vi "dataMerge.vi"(8 "error in (no error)":errorcluster, 10 "data":string[][][](array[string]), 11 "reference in":refnum<class "File Controller.lvclass">) -> (0 "error out":errorcluster, 3 "reference out":refnum<class "File Controller.lvclass">)   [LabVIEW 2015, in "File Controller.lvclass"]
uses:
  File Controller.lvclass
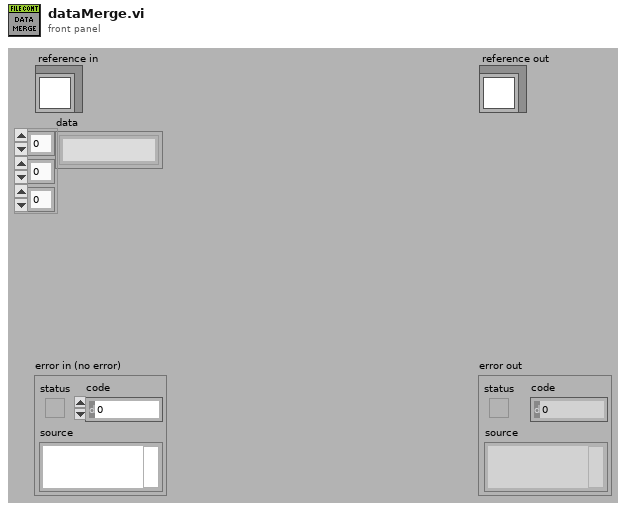
[diagram p1: front panel]
types:
  T1 = typedef "File Controller.lvclass/ObjectAttributesRef.ctl" = refnum<data-value>
  T2 = typedef "File Controller.lvclass/ObjectAttributes.ctl" = cluster{"MyAttribute":dbl, "file_path":path, "file_type":T3, "data":string[][][], "excel_file_ref":refnum<class "excelFile.lvclass">, "sheetName":string[], "subject_refs":refnum<class "subject.lvclass">[], "temp_data":string[][][]}
  T3 = typedef "excelFile.lvclass/fileType.ctl" = enum16{"database", "CosmedTest"}
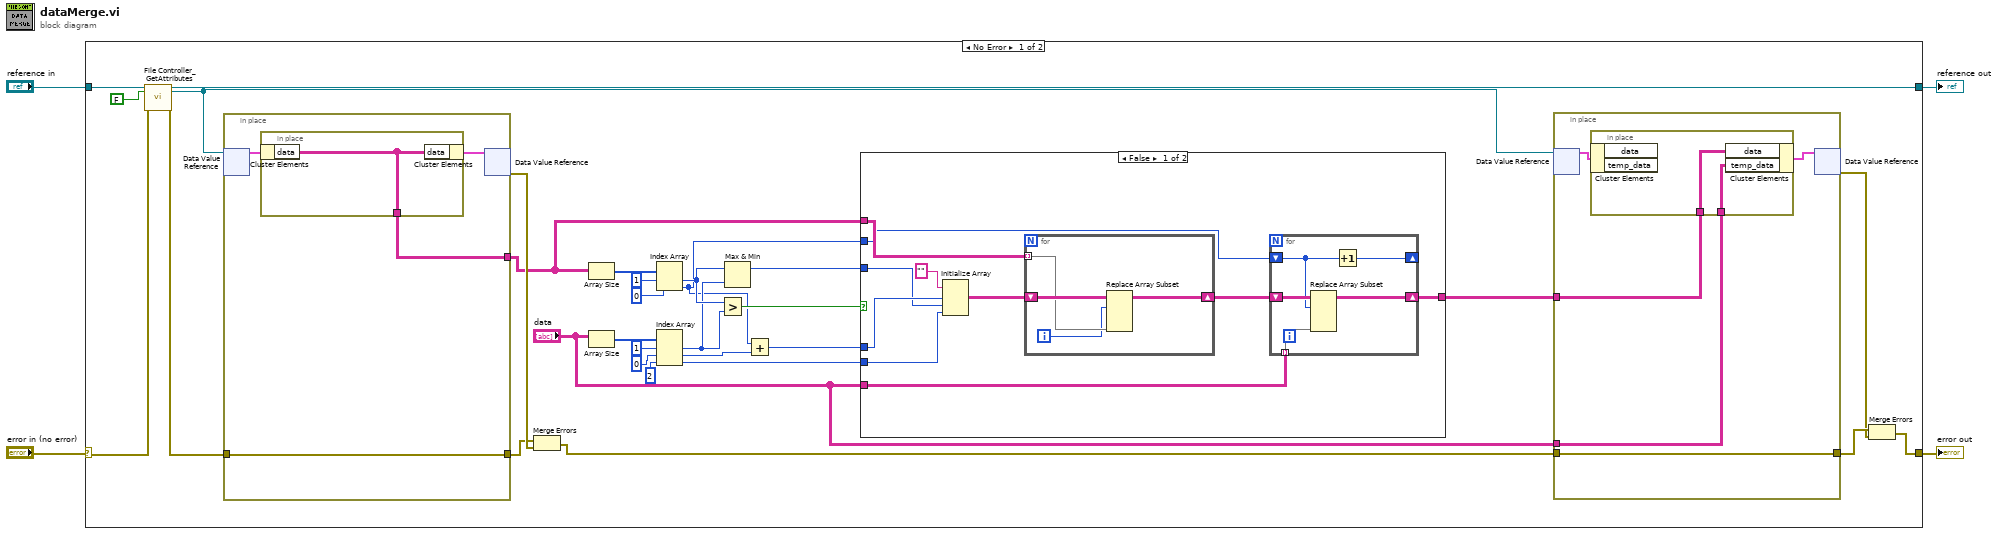
[diagram p0: block diagram]
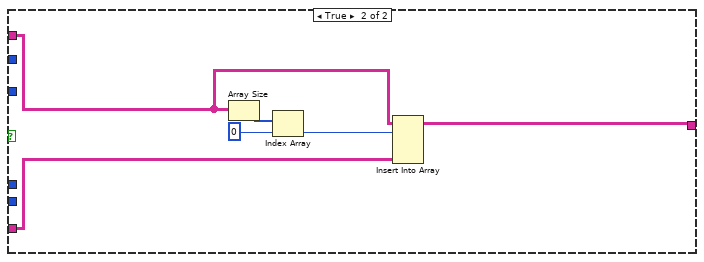
[diagram p2: hidden frame]
diagram:
  n1 = case shown="No Error" "error in (no error)" {
    selector: "error in (no error)" -> [w30 w73]
    tunnel: [w7 w73] -> w3
    tunnel: [w28 w72] -> w1
    tunnel: "reference in" -> [w32 w72]
    frame No Error {
      n2 = call "File Controller_GetAttributes.vi"("reference in"=w32, "return data? (T)"=FALSE, "error in (no error)"=w30) -> ("reference out"=w28:refnum<class "File Controller.lvclass">, "attributes ref"=w9:T1, "error out"=w29:errorcluster)  [unwired: 13 in, 1 out]
      n3 = in-place {
        in-place-border: w29 -> [w68]
        in-place-border: [w68] -> w33
        in-place-border: [w67] -> w22
        n4 = in-place-dvr #1(w9) -> (w69:T2)  [unwired: 1 out]
        n5 = in-place {
          in-place-border: [w71] -> w67
          n6 = in-place-cluster #2(w69) -> ("data"=w71:string[][][])
          n7 = in-place-cluster #2("data"=w71) -> (w70:T2)
        }
        n8 = in-place-dvr #1(w70) -> (w34:errorcluster)  [unwired: 1 out]
      }
      n9 = Merge Errors(w33, w34) -> (w11:errorcluster)
      n10 = Array Size(array=w22) -> (size(s)=w26:i32[])
      n11 = Array Size(array="data") -> (size(s)=w27:i32[])
      n12 = Index Array(array=w26, index #1=1 ("index"), index #2=0 ("index")) -> (element #1=w21:i32, element #2=w12:i32)
      n13 = Index Array(array=w27, index #1=1 ("index"), index #2=0 ("index"), index #3=2 ("index")) -> (element #1=w20:i32, element #2=w15:i32, element #3=w13:i32)
      n14 = Greater?(x=w21, y=w20) -> (0:w23:bool)
      n15 = Max & Min(x=w21, y=w20) -> (max(x,y)=w19:i32)  [unwired: 1 out]
      n16 = Add(x=w12, y=w15) -> (x+y=w14:i32)
      n17 = case shown="False" w23 {
        tunnel: w22 -> [w48 w66]
        tunnel: "data" -> [w46 w62]
        tunnel: w19 -> [w43 _]
        tunnel: w14 -> [w50 _]
        tunnel: w13 -> [w42 _]
        tunnel: w12 -> [w45 _]
        tunnel: [w44 w61] -> w10
        frame False {
          n18 = Initialize Array("", w50, w43, w42) -> (w49:string[][][])
          n19 = for {
            shift-right: [w59] -> w47
            shift-left: w49 -> [w60]
            tunnel: w48 -> [w58] mode=indexing
            i -> [w57]
            n20 = Replace Array Subset(array=w60, new element=w58, index (dim 0)=w57) -> (w59:string[][][])  [unwired: 2 in]
          }
          n21 = for {
            shift-right: [w55] -> w44
            shift-left: w47 -> [w56]
            tunnel: w46 -> [w54] mode=indexing
            shift-right: [w52] -> _
            shift-left: w45 -> [w53]
            n22 = Replace Array Subset(array=w56, new element=w54, index (dim 0)=w53) -> (w55:string[][][])  [unwired: 2 in]
            n23 = Increment(x=w53) -> (x+1=w52:i32)
          }
        }
        frame True {
          n24 = Array Size(array=w66) -> (size(s)=w65:i32[])
          n25 = Index Array(array=w65, index=0) -> (element=w63:i32)
          n26 = Insert Into Array(array=w66, index (dim 0)=w63, new element=w62) -> (w61:string[][][])  [unwired: 2 in]
        }
      }
      n27 = in-place {
        in-place-border: w11 -> [w37]
        in-place-border: [w37] -> w8
        in-place-border: w10 -> [w36]
        in-place-border: "data" -> [w35]
        n28 = in-place-dvr #3(w9) -> (w38:T2)  [unwired: 1 out]
        n29 = in-place {
          in-place-border: w36 -> [w41]
          in-place-border: w35 -> [w40]
          n30 = in-place-cluster #4(w38) -> ()  [unwired: 2 out]
          n31 = in-place-cluster #4("data"=w41, "temp_data"=w40) -> (w39:T2)
        }
        n32 = in-place-dvr #3(w39) -> (w6:errorcluster)  [unwired: 1 out]
      }
      n33 = Merge Errors(w8, w6) -> (w7:errorcluster)
    }
    frame Error {
    }
  }
  "error out" <- w3
  "reference out" <- w1
